vi "Parse Response String.vi"(8 "error in (no error)":errorcluster, 11 "Response String":string) -> (0 "error out":errorcluster, 3 "channelProperties":T1={"channel"=1, "gain"=enum."10", "input"=enum."SE+", "shunt"=enum."50", "couple"=enum."DC", "filter"=enum."ON"} {"channel" min=1 max=8 step=1})   [LabVIEW 2019, in "KH7008.lvlib"]
uses:
  KH7008.lvlib
  typedefs/channelProperties--Cluster.ctl
  typedefs/channel--numeric.ctl
  typedefs/gain--enum.ctl
  typedefs/Input--Enum.ctl
  typedefs/shunt--enum.ctl
  typedefs/couple--Enum.ctl
  typedefs/Filter--Enum.ctl
panel:
  # "CH2;G1;CP2;BW2;IC2;SR1"
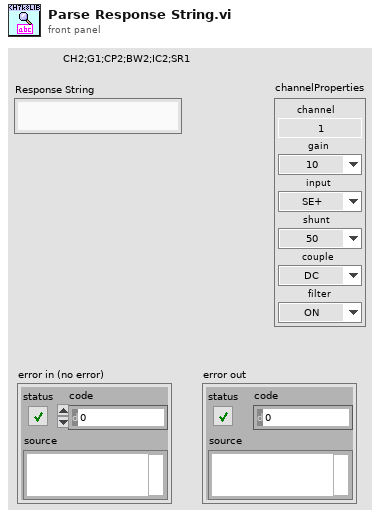
[diagram p1: front panel]
types:
  T1 = typedef "KH7008.lvlib/channelProperties--Cluster.ctl" = cluster{"channel":T2, "gain":T3, "input":T4, "shunt":T5, "couple":T6, "filter":T7}
  T2 = typedef "KH7008.lvlib/channel--numeric.ctl" = u16
  T3 = typedef "KH7008.lvlib/gain--enum.ctl" = enum16{"1", "10", "100", "1000"}
  T4 = typedef "KH7008.lvlib/input--enum.ctl" = enum16{"OFF", "SE+", "SE-", "DIFF"}
  T5 = typedef "KH7008.lvlib/shunt--enum.ctl" = enum16{"Open", "50", "500", "5k", "50k", "10M"}
  T6 = typedef "KH7008.lvlib/couple--enum.ctl" = enum16{"AC", "DC"}
  T7 = typedef "KH7008.lvlib/filter--enum.ctl" = enum16{"OFF", "ON"}
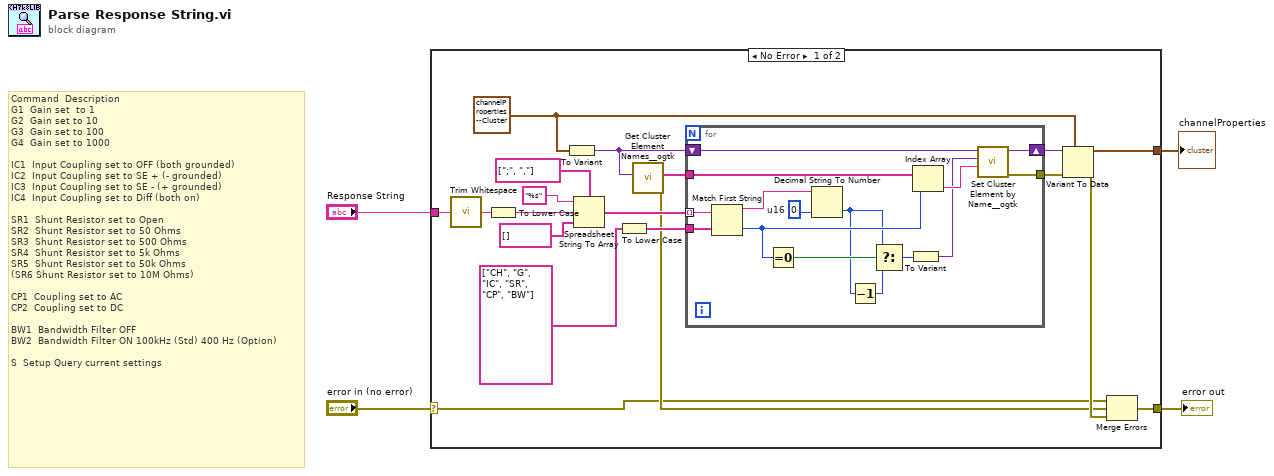
[diagram p0: block diagram]
diagram:
  # "Command  Description \nG1  Gain set  to 1 \nG2  Gain set to 10 \nG3  Gain set to 100 \nG4  Gain set to 1000 \n   \nIC1  Input Coupling set to OFF (both grounded) \nIC2  Input Coupling set to SE + (- grounded) \nIC3  Input Coupling set to SE - (+ grounded) \nIC4  Input Coupling set to Diff (both on) \n   \nSR1  Shunt Resistor set to Open \nSR2  Shunt Resistor set to 50 Ohms \nSR3  Shunt Resistor set to 500 Ohms \nSR4  Shunt Resistor set to 5k Ohms \nSR5  Shunt Resistor set to 50k Ohms \n(SR6 Shunt Resistor set to 10M Ohms)\n   \nCP1  Coupling set to AC \nCP2  Coupling set to DC \n   \nBW1  Bandwidth Filter OFF \nBW2  Bandwidth Filter ON 100kHz (Std) 400 Hz (Option)\n   \nS  Setup Query current settings"
  n1 = case shown="No Error" "error in (no error)" {
    selector: "error in (no error)" -> [w5 w39]
    tunnel: "Response String" -> [w23 _]
    tunnel: [w17 _] -> w3
    tunnel: [w15 w39] -> w2
    frame No Error {
      w7 = T1 {"channel"=1, "gain"=enum."10", "input"=enum."SE+", "shunt"=enum."50", "couple"=enum."DC", "filter"=enum."ON"} ("channelProperties")
      n2 = call <vilib>:"Trim Whitespace.vi"("string"=w23) -> ("trimmed string"=w22:string)  [unwired: 1 in]
      n3 = To Lower Case(string=w22) -> (all lower case string=w11:string)
      n4 = To Variant(anything=w7) -> (Variant=w20:variant)
      n5 = Spreadsheet String To Array(delimiter (Tab)=string[] [";", ","] ("delimiter"), format string="%s", spreadsheet string=w11, array type (2D Dbl)=string[] []) -> (array=w12:string[])
      n6 = To Lower Case(string=string[] ["CH", "G", "IC", "SR", "CP", "BW"] ("operators (none)")) -> (all lower case string=w14:string[])
      n7 = call <userlib>:"Get Cluster Element Names__ogtk.vi"("Cluster"=w20) -> ("error out"=w6:errorcluster, "Element Names"=w19:string[])  [unwired: 9 in]
      n8 = for {
        tunnel: w12 -> [w38] mode=indexing
        tunnel: w14 -> [w37]
        shift-right: [w35] -> w21
        shift-left: w20 -> [w36]
        tunnel: w19 -> [w33]
        tunnel: [w32] -> w18
        w29 = u16 0  # u16
        n9 = Match First String(2:w37, 3:w38) -> (0:w28:i32, 1:w30:string)
        n10 = Equal To 0?(x=w28) -> (x = 0?=w27:bool)
        n11 = Decimal String To Number(string=w30, default (0L)=w29) -> (number=w25:u16)  [unwired: 1 in, 1 out]
        n12 = Decrement(x=w25) -> (x-1=w24:u16)
        n13 = Select(t=w25, s=w27, f=w24) -> (s? t:f=w26:u16)
        n14 = To Variant(anything=w26) -> (Variant=w31:variant)
        n15 = Index Array(array=w33, index=w28) -> (element=w34:string)
        n16 = call <userlib>:"Set Cluster Element by Name__ogtk.vi"("Element Name (\"\": New Element Data Name)"=w34, "New Element Value"=w31, "Cluster"=w36) -> ("error out"=w32:errorcluster, "VCluster out"=w35:variant)  [unwired: 6 in, 1 out]
      }
      n17 = Variant To Data(error in=w18, type=w7, Variant=w21) -> (data=w17:T1, error out=w16:errorcluster)
      n18 = Merge Errors(w5, w6, w16) -> (w15:errorcluster)
    }
    frame Error {
    }
  }
  "error out" <- w2
  "channelProperties" <- w3
